vi "RCServo All Events Example.vi"() -> ()   [LabVIEW 2012, in "Phidget RC Servo.lvlib"]
uses:
  <instrlib>/Phidgets/Phidget RC Servo/Phidget RC Servo.lvlib
  <instrlib>/Phidgets/Phidget RC Servo/Public/RCServoStart.vi
  <instrlib>/Phidgets/Phidget RC Servo/Public/RCServoClose.vi
  <instrlib>/Phidgets/Phidget Common/Phidget Common.lvlib
panel:
  in  "stop 3":bool caption="stop"
  in  "stop 2":bool caption="stop"
  in  "stop":bool
  in  "RCServo Initialization Data":T1={"Velocity Limit"=180.0, "Acceleration"=360.0, "Min PW"=550, "Max PW"=2350, "Max Position"=180.0, "Min Position"=0.0, "Speed Ramping State"=TRUE}
  out "Velocity":dbl format="%.2f"
  out "Current Position":dbl format="%.2f"
  out "Position Reached":dbl format="%.2f"
  out "Serial Number Return":i32
  in  "Device Info":T2={"Serial Number"=-1, "Channel"=0, "Port"=0}
  out "error out":errorcluster
  # "Be sure to use this stop button to stop the program.\nIf you use the \"Abort Execution\" button, you will\nneed to use PhidgetResetLibrary.vi or restart Labview \nin order for any Phidgets to work."
  # "Enabled\n\nDisabled"
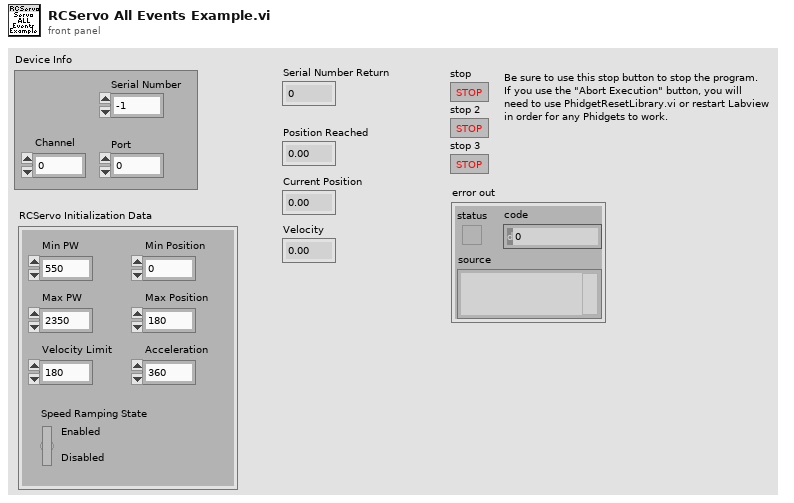
[diagram p1: front panel]
types:
  T1 = cluster{"Velocity Limit":dbl, "Acceleration":dbl, "Min PW":i32, "Max PW":i32, "Max Position":dbl, "Min Position":dbl, "Speed Ramping State":bool}
  T2 = cluster{"Serial Number":i32, "Channel":i32, "Port":i32}
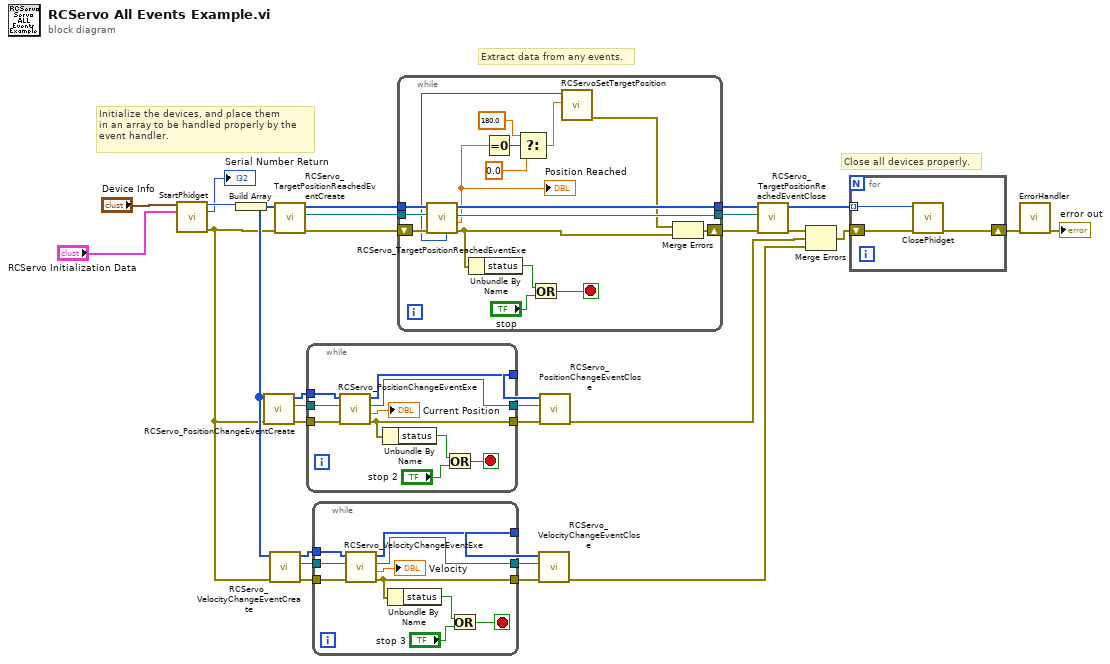
[diagram p0: block diagram]
diagram:
  # "Close all devices properly."
  # "Extract data from any events."
  # "Initialize the devices, and place them\nin an array to be handled properly by the\nevent handler."
  n1 = call-poly <instrlib>:"StartPhidget.vi"("Device Info"="Device Info", "RCServo Initialization Data"="RCServo Initialization Data") -> ("Phidget ID"=w23:u64, "Serial Number Return"=→"Serial Number Return":i32, "error out"=w2:errorcluster)  [unwired: 10 in, 1 out]
  n2 = Build Array(w23) -> (w22:u64[])
  n3 = call <instrlib>:"RCServo_PositionChangeEventCreate.vi"("error in (no error)"=w2, "Devices In"=w22) -> ("error out"=w16:errorcluster, "Event Registration Refnum"=w18:refnum<event-registration>, "Devices Out"=w19:u64[])  [unwired: 7 in]
  n4 = call <instrlib>:"RCServo_VelocityChangeEventCreate.vi"("error in (no error)"=w2, "Devices In"=w22) -> ("error out"=w17:errorcluster, "Event Registration Refnum"=w13:refnum<event-registration>, "Devices Out"=w12:u64[])  [unwired: 7 in]
  n5 = call <instrlib>:"RCServo_TargetPositionReachedEventCreate.vi"("error in (no error)"=w2, "Devices In"=w22) -> ("error out"=w4:errorcluster, "Event Registration Refnum"=w30:refnum<event-registration>, "Devices Out"=w31:u64[])  [unwired: 7 in]
  n6 = while {
    tunnel: w19 -> [w41]
    tunnel: w18 -> [w40]
    tunnel: w16 -> [w39]
    tunnel: [w32] -> w15
    tunnel: [w37] -> w11
    tunnel: [w36] -> w10
    stop <- w33 stop-if-true
    n7 = call <instrlib>:"RCServo_PositionChangeEventExe.vi"("error in (no error)"=w39, "Event Registration Refnum In"=w40, "Devices In"=w41) -> ("error out"=w32:errorcluster, "Position"=→"Current Position":dbl, "Event Registration Refnum Out"=w37:refnum<event-registration>, "Devices Out"=w36:u64[])  [unwired: 2 in, 3 out]
    n8 = Unbundle By Name(w32) -> ("status"=w34:bool)
    n9 = Or(x=w34, y="stop 2") -> (x .or. y?=w33:bool)
  }
  n10 = while {
    tunnel: w17 -> [w51]
    tunnel: [w42] -> w14
    tunnel: w13 -> [w50]
    tunnel: w12 -> [w49]
    tunnel: [w48] -> w9
    tunnel: [w47] -> w8
    stop <- w43 stop-if-true
    n11 = call <instrlib>:"RCServo_VelocityChangeEventExe.vi"("error in (no error)"=w51, "Event Registration Refnum In"=w50, "Devices In"=w49) -> ("error out"=w42:errorcluster, "Velocity"=→"Velocity":dbl, "Event Registration Refnum Out"=w48:refnum<event-registration>, "Devices Out"=w47:u64[])  [unwired: 2 in, 3 out]
    n12 = Unbundle By Name(w42) -> ("status"=w44:bool)
    n13 = Or(x=w44, y="stop 3") -> (x .or. y?=w43:bool)
  }
  n14 = while {
    tunnel: w31 -> [w68]
    tunnel: w30 -> [w65]
    tunnel: [w67] -> w27
    shift-right: [w63] -> w21
    shift-left: w4 -> [w62]
    tunnel: [w66] -> w24
    stop <- w59 stop-if-true
    n15 = call <instrlib>:"RCServo_TargetPositionReachedEventExe.vi"("error in (no error)"=w62, "Event Registration Refnum In"=w65, "Devices In"=w68) -> ("error out"=w64:errorcluster, "Position"=w52:dbl, "Event Registration Refnum Out"=w67:refnum<event-registration>, "Devices Out"=w66:u64[], "phid"=w53:u64)  [unwired: 2 in, 2 out]
    "Position Reached" <- w52
    n16 = Unbundle By Name(w64) -> ("status"=w60:bool)
    n17 = Equal To 0?(x=w52) -> (x = 0?=w58:bool)
    n18 = Select(t=180.0, s=w58, f=0.0) -> (s? t:f=w55:dbl)
    n19 = Or(x=w60, y="stop") -> (x .or. y?=w59:bool)
    n20 = call <instrlib>:"RCServoSetTargetPosition.vi"("Target Position"=w55, "Device In"=w53) -> ("error out"=w54:errorcluster)  [unwired: 7 in, 1 out]
    n21 = Merge Errors(w54, w64) -> (w63:errorcluster)
  }
  n22 = call <instrlib>:"RCServo_VelocityChangeEventClose.vi"("error in (no error)"=w14, "Event Registration Refnum In"=w9, "Devices In"=w8) -> ("error out"=w5:errorcluster)  [unwired: 7 in, 1 out]
  n23 = call <instrlib>:"RCServo_PositionChangeEventClose.vi"("error in (no error)"=w15, "Event Registration Refnum In"=w11, "Devices In"=w10) -> ("error out"=w6:errorcluster)  [unwired: 7 in, 1 out]
  n24 = call <instrlib>:"RCServo_TargetPositionReachedEventClose.vi"("error in (no error)"=w21, "Event Registration Refnum In"=w27, "Devices In"=w24) -> ("error out"=w7:errorcluster, "Devices Out"=w25:u64[])  [unwired: 7 in]
  n25 = Merge Errors(w7, w6, w5) -> (w3:errorcluster)
  n26 = for {
    tunnel: w25 -> [w69] mode=indexing
    shift-right: [w71] -> w29
    shift-left: w3 -> [w70]
    n27 = call-poly <instrlib>:"ClosePhidget.vi"("error in"=w70, "Device In"=w69) -> ("error out"=w71:errorcluster)  [unwired: 9 in]
  }
  n28 = call <instrlib>:"ErrorHandler.vi"("error in"=w29) -> ("error out"=→"error out":errorcluster)  [unwired: 9 in, 1 out]
